vi "Process Asynch.vi"(11 "IO in":refnum<class "IO.lvclass">) -> (3 "IO out":refnum<class "IO.lvclass">)   [LabVIEW 2021, in "IO.lvclass"]
uses:
  IO.lvclass
  IO.lvclass/IO.ctl
  Memory Map/Memory Map.lvclass
  Memory/Memory.lvclass
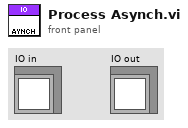
[diagram p1: front panel]
types:
  T1 = typedef "Memory Map.lvclass/Active Device.ctl" = enum16{"Error", "None", "RAM", "EEPROM", "VIA"}
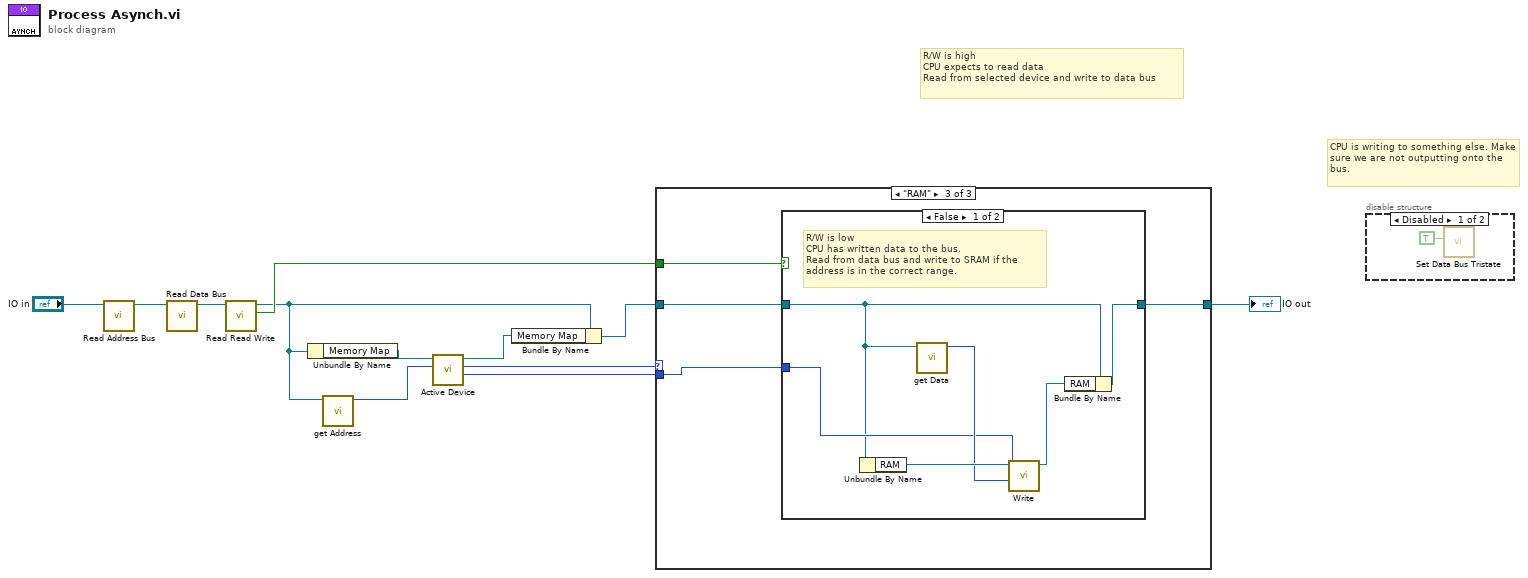
[diagram p0: block diagram]
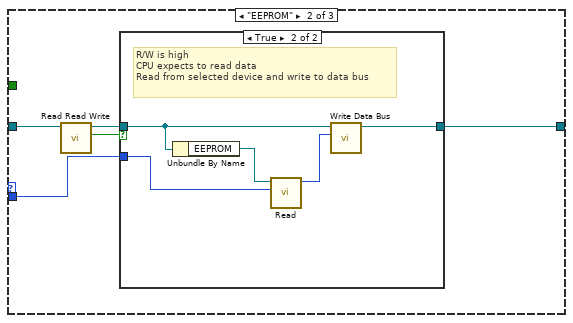
[diagram p4: hidden frame]
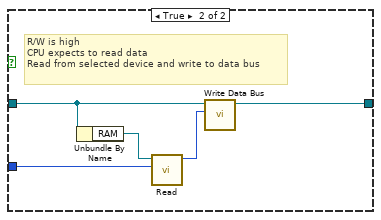
[diagram p6: hidden frame]
diagram:
  # "CPU is writing to something else. Make sure we are not outputting onto the bus."
  # "R/W is high\nCPU expects to read data\nRead from selected device and write to data bus"
  n1 = call "Read Address Bus.vi"("IO in"="IO in") -> ("IO out"=w8:refnum<class "IO.lvclass">)  [unwired: 9 in, 1 out]
  n2 = call "Read Data Bus.vi"("IO in"=w8) -> ("IO out"=w7:refnum<class "IO.lvclass">)  [unwired: 9 in, 1 out]
  n3 = call "Read Read Write.vi"("IO in"=w7) -> ("R/W"=w6:bool, "IO out"=w3:refnum<class "IO.lvclass">)  [unwired: 8 in, 1 out]
  n4 = Unbundle By Name(w3) -> ("Memory Map"=w10:refnum<class "Memory Map.lvclass">)
  n5 = call "get Address.vi"("IO in"=w3) -> ("Address"=w11:u16)  [unwired: 10 in]
  n6 = call "Active Device.vi"("Address"=w11, "Memory Map in"=w10) -> ("Relative Address"=w5:u16, "Active Device"=w4:T1, "Memory Map out"=w1:refnum<class "Memory Map.lvclass">)  [unwired: 7 in]
  n7 = Bundle By Name(cluster=w3, "Memory Map"=w1) -> (w2:refnum<class "IO.lvclass">)
  n8 = case shown="\"RAM\"" w4 {
    tunnel: [w13 w18 w28] -> w12
    tunnel: w2 -> [w13 w15 w26]
    tunnel: w5 -> [_ w17 w27]
    tunnel: w6 -> [_ _ w25]
    frame Default {
    }
    frame "EEPROM" {
      n9 = call "Read Read Write.vi"("IO in"=w15) -> ("R/W"=w14:bool, "IO out"=w16:refnum<class "IO.lvclass">)  [unwired: 8 in, 1 out]
      n10 = case shown="True" w14 {
        tunnel: [w19 w24] -> w18
        tunnel: w17 -> [_ w21]
        tunnel: w16 -> [w19 w20]
        frame False {
        }
        frame True {
          # "R/W is high\nCPU expects to read data\nRead from selected device and write to data bus"
          n11 = Unbundle By Name(w20) -> ("EEPROM"=w22:refnum<class "Memory.lvclass">)
          n12 = call "Read.vi"("Address"=w21, "Memory in"=w22) -> ("Data"=w23:u8)  [unwired: 9 in]
          n13 = call "Write Data Bus.vi"("Data"=w23, "IO in"=w20) -> ("IO out"=w24:refnum<class "IO.lvclass">)  [unwired: 8 in, 1 out]
        }
      }
    }
    frame "RAM" {
      n14 = case shown="False" w25 {
        tunnel: [w31 w39] -> w28
        tunnel: w27 -> [w32 w36]
        tunnel: w26 -> [w29 w35]
        frame False {
          # "R/W is low\nCPU has written data to the bus. \nRead from data bus and write to SRAM if the address is in the correct range."
          n15 = Unbundle By Name(w29) -> ("RAM"=w34:refnum<class "Memory.lvclass">)
          n16 = call "get Data.vi"("IO in"=w29) -> ("Data"=w33:u8)  [unwired: 10 in]
          n17 = call "Write.vi"("Data"=w33, "Address"=w32, "Memory in"=w34) -> ("Memory out"=w30:refnum<class "Memory.lvclass">)  [unwired: 8 in]
          n18 = Bundle By Name(cluster=w29, "RAM"=w30) -> (w31:refnum<class "IO.lvclass">)
        }
        frame True {
          # "R/W is high\nCPU expects to read data\nRead from selected device and write to data bus"
          n19 = Unbundle By Name(w35) -> ("RAM"=w37:refnum<class "Memory.lvclass">)
          n20 = call "Read.vi"("Address"=w36, "Memory in"=w37) -> ("Data"=w38:u8)  [unwired: 9 in]
          n21 = call "Write Data Bus.vi"("Data"=w38, "IO in"=w35) -> ("IO out"=w39:refnum<class "IO.lvclass">)  [unwired: 8 in, 1 out]
        }
      }
    }
  }
  "IO out" <- w12
  n22 = disable-structure shown="Disabled" {
    frame Disabled {
      n23 = call "Set Data Bus Tristate.vi"("Tristate"=TRUE) -> ()  [unwired: 9 in, 2 out]
    }
    frame Enabled {
    }
  }
